vi "Stepper FPGA.vi"() -> ()   [LabVIEW 2017]
uses:
  <vilib>/rvi/Emulation/niFpgaGetClockAttributes.vi
  <vilib>/rvi/Emulation/niFpgaSctlEmulationGetInTimedLoop.vi
  <vilib>/rvi/Emulation/niFpgaEmulationReportErrorSimple.vi
  <vilib>/rvi/eio/common/nirviEmuTemplateMethod_errors.vi
  <vilib>/rvi/Emulation/niFpgaCriticalErrorInLSC.vi
  <vilib>/eio/EIONode/EIONode.xnode
panel:
  out "Cluster":cluster{i16, i16, i16, i16, i16, i16, i16, i16}
  in  "Skipper":cluster{i16, i16, i16, i16, i16, i16, i16, i16}
  in  "Steps":cluster{i16, i16, i16, i16, i16, i16, i16, i16}
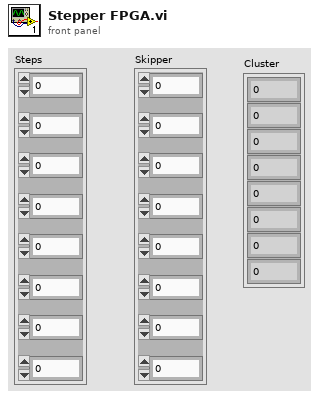
[diagram p1: front panel]
types:
  T1 = cluster{bool, bool, bool, bool, bool, bool, bool, bool}
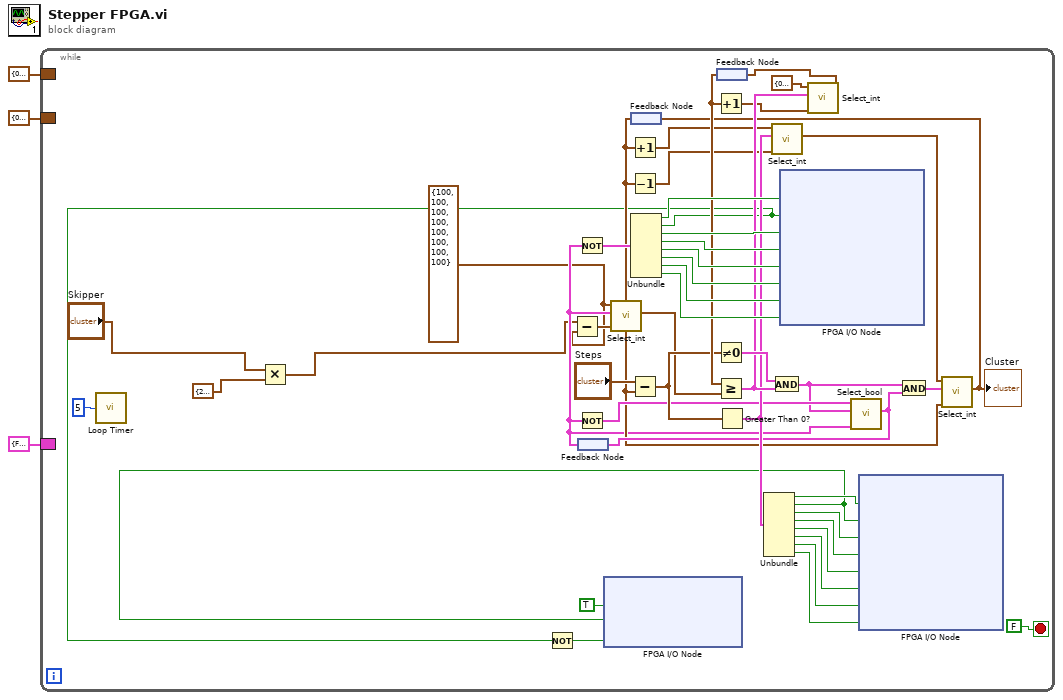
[diagram p0: block diagram]
diagram:
  n1 = while {
    border: T1 {FALSE, FALSE, FALSE, FALSE, FALSE, FALSE, FALSE, FALSE} -> [_]
    border: cluster{i16, i16, i16, i16, i16, i16, i16, i16} {0, 0, 0, 0, 0, 0, 0, 0} -> [_]
    border: cluster{i16, i16, i16, i16, i16, i16, i16, i16} {0, 0, 0, 0, 0, 0, 0, 0} ("output cluster") -> [_]
    stop <- FALSE stop-if-true
    w7 = cluster{i16, i16, i16, i16, i16, i16, i16, i16} {100, 100, 100, 100, 100, 100, 100, 100} ("True")
    n2 = call "Loop Timer"("Count(uSec)"=u32 5) -> ()  [unwired: 1 out]
    n3 = Multiply(x="Skipper", y=cluster{i16, i16, i16, i16, i16, i16, i16, i16} {2, 2, 2, 2, 2, 2, 2, 2}) -> (x*y=w5:cluster{i16, i16, i16, i16, i16, i16, i16, i16})
    n4 = Subtract(x=w5, y=w7) -> (x-y=w8:cluster{i16, i16, i16, i16, i16, i16, i16, i16})
    n5 = feedback #1() -> (w14:T1)
    n6 = Not(x=w14) -> (.not. x?=w39:T1)
    n7 = Not(x=w14) -> (.not. x?=w21:T1)
    n8 = call "Select_int.vi"("False"=w8, "Input"=w14, "True"=w7) -> ("output"=w13:cluster{i16, i16, i16, i16, i16, i16, i16, i16})  [unwired: 8 in]
    n9 = feedback #2() -> (w18:cluster{i16, i16, i16, i16, i16, i16, i16, i16})
    n10 = Increment(x=w18) -> (x+1=w17:cluster{i16, i16, i16, i16, i16, i16, i16, i16})
    n11 = Decrement(x=w18) -> (x-1=w16:cluster{i16, i16, i16, i16, i16, i16, i16, i16})
    n12 = Subtract(x="Steps", y=w18) -> (x-y=w29:cluster{i16, i16, i16, i16, i16, i16, i16, i16})
    n13 = Unbundle(w39) -> (w40:bool, w10:bool, w49:bool, w48:bool, w47:bool, w46:bool, w45:bool, w44:bool)
    n14 = Not(x=w10) -> (.not. x?=w11:bool)
    n15 = Not Equal To 0?(x=w29) -> (x != 0?=w42:T1)
    n16 = feedback #3() -> (w37:cluster{i16, i16, i16, i16, i16, i16, i16, i16})
    n17 = Increment(x=w37) -> (x+1=w27:cluster{i16, i16, i16, i16, i16, i16, i16, i16})
    n18 = Greater Or Equal?(x=w37, y=w13) -> (x >= y?=w28:T1)
    n19 = Greater Than 0?(x=w29) -> (x > 0?=w24:T1)
    n20 = Unbundle(w24) -> (w30:bool, w9:bool, w36:bool, w35:bool, w34:bool, w33:bool, w32:bool, w31:bool)
    n21 = xnode "FPGA I/O Node"("ConnectorC/DIO0"=TRUE, "ConnectorC/DIO1"=w9, "ConnectorC/DIO2"=w11) -> ()  [unwired: 3 in, 3 out]
    n22 = call "Select_int.vi"("False"=w16, "Input"=w24, "True"=w17) -> ("output"=w23:cluster{i16, i16, i16, i16, i16, i16, i16, i16})  [unwired: 8 in]
    n23 = And(x=w42, y=w28) -> (x .and. y?=w20:T1)
    n24 = xnode "FPGA I/O Node"("ConnectorA/DIO0"=w40, "ConnectorA/DIO2"=w10, "ConnectorA/DIO11"=w49, "ConnectorA/DIO5"=w48, "ConnectorA/DIO6"=w47, "ConnectorA/DIO13"=w46, "ConnectorA/DIO9"=w45, "ConnectorA/DIO14"=w44) -> ()  [unwired: 8 in, 8 out]
    n25 = call "Select_int.vi"("False"=w27, "Input"=w28, "True"=cluster{i16, i16, i16, i16, i16, i16, i16, i16} {0, 0, 0, 0, 0, 0, 0, 0}) -> ("output"=w26:cluster{i16, i16, i16, i16, i16, i16, i16, i16})  [unwired: 8 in]
    n26 = feedback-in #3(w26) -> ()
    n27 = call "Select_bool.vi"("False"=w14, "Input"=w20, "True"=w21) -> ("output cluster"=w19:T1)  [unwired: 8 in]
    n28 = feedback-in #1(w19) -> ()
    n29 = xnode "FPGA I/O Node"("ConnectorA/DIO1"=w30, "ConnectorA/DIO3"=w9, "ConnectorA/DIO4"=w36, "ConnectorA/DIO12"=w35, "ConnectorA/DIO7"=w34, "ConnectorA/DIO8"=w33, "ConnectorA/DIO10"=w32, "ConnectorA/DIO15"=w31) -> ()  [unwired: 8 in, 8 out]
    n30 = And(x=w20, y=w19) -> (x .and. y?=w22:T1)
    n31 = call "Select_int.vi"("False"=w18, "Input"=w22, "True"=w23) -> ("output"=w15:cluster{i16, i16, i16, i16, i16, i16, i16, i16})  [unwired: 8 in]
    "Cluster" <- w15
    n32 = feedback-in #2(w15) -> ()
  }
